vi "4 Bits Read.vi"(6 "E?E1:E2 (E1)":bool=TRUE, 9 "RS":bool, 11 "device connection map":T1={"RS"="RS", "R/W"="RW", "E1"="E1", "E2"="E2", "DB4"="DB4", "DB5"="DB5", "DB6"="DB6", "DB7"="DB7"}) -> (1 "value":u8)   [LabVIEW 2017, in "HD44780 FPGA.lvlib"]
uses:
  HD44780 FPGA.lvlib
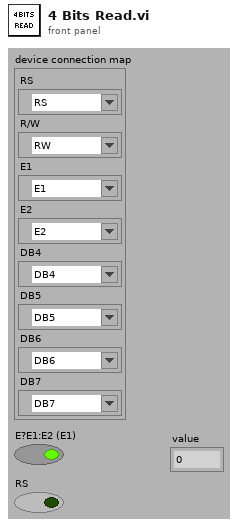
[diagram p1: front panel]
types:
  T1 = cluster{"RS":refnum<k21>, "R/W":refnum<k21>, "E1":refnum<k21>, "E2":refnum<k21>, "DB4":refnum<k21>, "DB5":refnum<k21>, "DB6":refnum<k21>, "DB7":refnum<k21>}
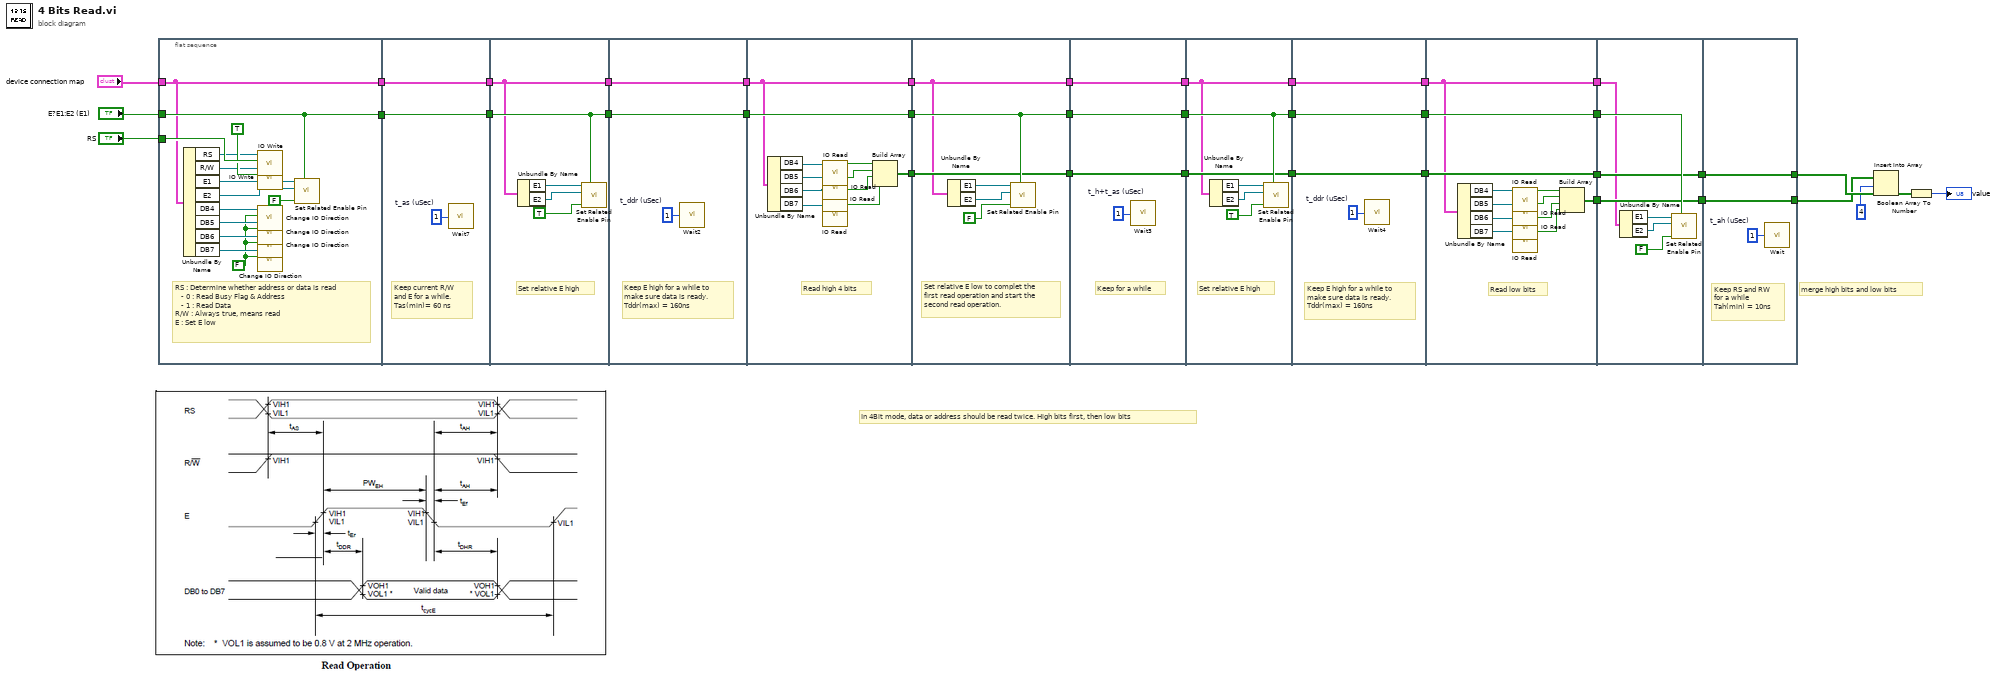
[diagram p0: block diagram]
diagram:
  # "merge high bits and low bits"
  # "In 4Bit mode, data or address should be read twice. High bits first, then low bits"
  n1 = flat-sequence {
    tunnel: "RS" -> [w51]
    tunnel: "E?E1:E2 (E1)" -> [w39]
    tunnel: "device connection map" -> [w38]
    tunnel: [w39] -> w7
    tunnel: [w38] -> w6
    tunnel: [w53] -> w30
    tunnel: [w52] -> w15
    tunnel: w7 -> [w53]
    tunnel: w6 -> [w52]
    tunnel: w30 -> [w58]
    tunnel: [w58] -> w29
    tunnel: [w57] -> w16
    tunnel: w15 -> [w57]
    tunnel: w29 -> [w61]
    tunnel: [w61] -> w28
    tunnel: w16 -> [w60]
    tunnel: [w60] -> w14
    tunnel: [w73] -> w5
    tunnel: w28 -> [w68]
    tunnel: [w68] -> w4
    tunnel: [w63] -> w3
    tunnel: w14 -> [w63]
    tunnel: w5 -> [w77]
    tunnel: [w77] -> w27
    tunnel: w4 -> [w79]
    tunnel: [w79] -> w26
    tunnel: [w76] -> w13
    tunnel: w3 -> [w76]
    tunnel: w27 -> [w82]
    tunnel: [w82] -> w25
    tunnel: w26 -> [w81]
    tunnel: [w81] -> w24
    tunnel: w13 -> [w80]
    tunnel: [w80] -> w11
    tunnel: w25 -> [w87]
    tunnel: [w87] -> w23
    tunnel: w24 -> [w88]
    tunnel: [w88] -> w22
    tunnel: [w86] -> w12
    tunnel: w11 -> [w86]
    tunnel: w23 -> [w92]
    tunnel: [w92] -> w21
    tunnel: w22 -> [w91]
    tunnel: [w91] -> w20
    tunnel: w12 -> [w90]
    tunnel: [w90] -> w10
    tunnel: w21 -> [w100]
    tunnel: [w100] -> w19
    tunnel: [w101] -> w18
    tunnel: w20 -> [w99]
    tunnel: [w99] -> w17
    tunnel: w10 -> [w94]
    tunnel: [w94] -> w9
    tunnel: w19 -> [w110]
    tunnel: w18 -> [w109]
    tunnel: w17 -> [w112]
    tunnel: w9 -> [w108]
    tunnel: [w110] -> w2
    tunnel: [w109] -> w1
    tunnel: [w114] -> w31
    tunnel: [w115] -> w36
    tunnel: w2 -> [w115]
    tunnel: w1 -> [w114]
    frame #0 {
      w40 = FALSE ("T? write:read")
      # "RS : Determine whether address or data is read\n   - 0 : Read Busy Flag & Address  \n   - 1 : Read Data\nR/W : Always true, means read\nE : Set E low"
      n2 = Unbundle By Name(w38) -> ("RS"=w49:refnum<k21>, "R/W"=w48:refnum<k21>, "E1"=w47:refnum<k21>, "E2"=w46:refnum<k21>, "DB4"=w44:refnum<k21>, "DB5"=w42:refnum<k21>, "DB6"=w41:refnum<k21>, "DB7"=w43:refnum<k21>)
      n3 = call "IO Write.vi"("data"=w51, "I/O"=w49) -> ()  [unwired: 10 in]
      n4 = call "IO Write.vi"("data"=TRUE, "I/O"=w48) -> ()  [unwired: 10 in]
      n5 = call "Change IO Direction.vi"("T? write:read"=w40, "I/O"=w44) -> ()  [unwired: 10 in]
      n6 = call "Change IO Direction.vi"("T? write:read"=w40, "I/O"=w42) -> ()  [unwired: 10 in]
      n7 = call "Change IO Direction.vi"("T? write:read"=w40, "I/O"=w41) -> ()  [unwired: 10 in]
      n8 = call "Change IO Direction.vi"("T? write:read"=w40, "I/O"=w43) -> ()  [unwired: 10 in]
      n9 = call "Set Related Enable Pin.vi"("E?E1:E2"=w39, "data"=FALSE, "E2"=w46, "E1"=w47) -> ()  [unwired: 8 in]
    }
    frame #1 {
      w54 = u8 1  # t_as (uSec)
      # "Keep current R/W \nand E for a while.\nTas(min)= 60 ns"
      n10 = call "Wait7"("Count(uSec)"=w54) -> ()  [unwired: 1 out]
    }
    frame #2 {
      # "Set relative E high"
      n11 = Unbundle By Name(w57) -> ("E1"=w56:refnum<k21>, "E2"=w55:refnum<k21>)
      n12 = call "Set Related Enable Pin.vi"("E?E1:E2"=w58, "data"=TRUE, "E2"=w55, "E1"=w56) -> ()  [unwired: 8 in]
    }
    frame #3 {
      w62 = u8 1  # t_ddr (uSec)
      # "Keep E high for a while to\nmake sure data is ready. \nTddr(max) = 160ns"
      n13 = call "Wait2"("Count(uSec)"=w62) -> ()  [unwired: 1 out]
    }
    frame #4 {
      # "Read high 4 bits"
      n14 = Unbundle By Name(w63) -> ("DB4"=w67:refnum<k21>, "DB5"=w66:refnum<k21>, "DB6"=w65:refnum<k21>, "DB7"=w64:refnum<k21>)
      n15 = call "IO Read.vi"("I/O"=w65) -> ("data"=w70:bool)  [unwired: 10 in]
      n16 = call "IO Read.vi"("I/O"=w64) -> ("data"=w69:bool)  [unwired: 10 in]
      n17 = call "IO Read.vi"("I/O"=w67) -> ("data"=w72:bool)  [unwired: 10 in]
      n18 = call "IO Read.vi"("I/O"=w66) -> ("data"=w71:bool)  [unwired: 10 in]
      n19 = Build Array(w72, w71, w70, w69) -> (w73:bool[])
    }
    frame #5 {
      # "Set relative E low to complet the\nfirst read operation and start the\nsecond read operation."
      n20 = Unbundle By Name(w76) -> ("E1"=w75:refnum<k21>, "E2"=w74:refnum<k21>)
      n21 = call "Set Related Enable Pin.vi"("E?E1:E2"=w79, "data"=FALSE, "E2"=w74, "E1"=w75) -> ()  [unwired: 8 in]
    }
    frame #6 {
      w83 = u8 1  # t_h+t_as (uSec)
      # "Keep for a while"
      n22 = call "Wait3"("Count(uSec)"=w83) -> ()  [unwired: 1 out]
    }
    frame #7 {
      # "Set relative E high"
      n23 = Unbundle By Name(w86) -> ("E1"=w85:refnum<k21>, "E2"=w84:refnum<k21>)
      n24 = call "Set Related Enable Pin.vi"("E?E1:E2"=w88, "data"=TRUE, "E2"=w84, "E1"=w85) -> ()  [unwired: 8 in]
    }
    frame #8 {
      w93 = u8 1  # t_ddr (uSec)
      # "Keep E high for a while to\nmake sure data is ready.\nTddr(max) = 160ns"
      n25 = call "Wait4"("Count(uSec)"=w93) -> ()  [unwired: 1 out]
    }
    frame #9 {
      # "Read low bits"
      n26 = Unbundle By Name(w94) -> ("DB4"=w98:refnum<k21>, "DB5"=w97:refnum<k21>, "DB6"=w96:refnum<k21>, "DB7"=w95:refnum<k21>)
      n27 = call "IO Read.vi"("I/O"=w98) -> ("data"=w105:bool)  [unwired: 10 in]
      n28 = call "IO Read.vi"("I/O"=w97) -> ("data"=w104:bool)  [unwired: 10 in]
      n29 = call "IO Read.vi"("I/O"=w96) -> ("data"=w103:bool)  [unwired: 10 in]
      n30 = call "IO Read.vi"("I/O"=w95) -> ("data"=w102:bool)  [unwired: 10 in]
      n31 = Build Array(w105, w104, w103, w102) -> (w101:bool[])
    }
    frame #10 {
      n32 = Unbundle By Name(w108) -> ("E1"=w107:refnum<k21>, "E2"=w106:refnum<k21>)
      n33 = call "Set Related Enable Pin.vi"("E?E1:E2"=w112, "data"=FALSE, "E2"=w106, "E1"=w107) -> ()  [unwired: 8 in]
    }
    frame #11 {
      w113 = u8 1  # t_ah (uSec)
      # "Keep RS and RW\nfor a while\nTah(min) = 10ns"
      n34 = call "Wait"("Count(uSec)"=w113) -> ()  [unwired: 1 out]
    }
  }
  n35 = Insert Into Array(array=w31, index=4, new element=w36) -> (w34:bool[])
  n36 = Boolean Array To Number(Boolean array=w34) -> (number=→"value":u8)
